vi "test.vi"() -> ()   [LabVIEW 2016]
panel:
  in  "布尔":bool
  in  "选项卡控件":enum32{"选项卡 1", "选项卡 2"}(tab)
  in  "数值 3":dbl
  out "数值":dbl
  out "数值 2":dbl
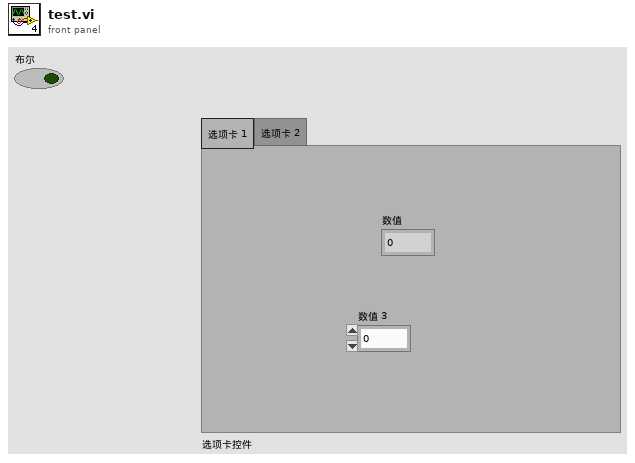
[diagram p1: front panel]
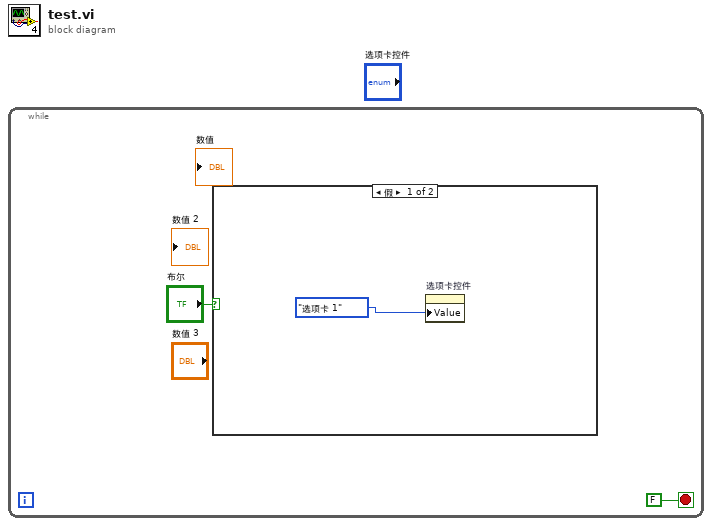
[diagram p0: block diagram]
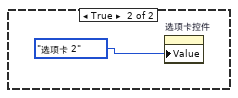
[diagram p2: hidden frame]
diagram:
  n1 = while {
    stop <- FALSE stop-if-true
    n2 = case shown="假" "布尔" {
      frame False {
        n3 = property on="选项卡控件" class="TabCtl (严格)"("Value"=enum32{"选项卡 1", "选项卡 2"}."选项卡 1" ("选项卡控件")) -> ()  [unwired: 2 in, 2 out]
      }
      frame True {
        n4 = property on="选项卡控件" class="TabCtl (严格)"("Value"=enum32{"选项卡 1", "选项卡 2"}."选项卡 2" ("选项卡控件")) -> ()  [unwired: 2 in, 2 out]
      }
    }
  }
